vi "PH_gentec_Powermeter.Action open connection.vi"(0 "VI in":refnum<vi>, 5 "error in (no error)":errorcluster) -> (14 "VI out":refnum<vi>, 19 "error out":errorcluster)   [LabVIEW 2014, in "PH_gentec_Powermeter.lvlib"]
uses:
  PH_gentec_Powermeter.lvlib
  PH_Powermeter_BaseClass/PH_Powermeter_BaseClass.State.ctl
  PH_Powermeter_BaseClass/PH_Powermeter_BaseClass.lvlib
  non_GPL/instr.lib/gentec-SOLO-PE/gentec-SOLO-PE - Driver.lvlib
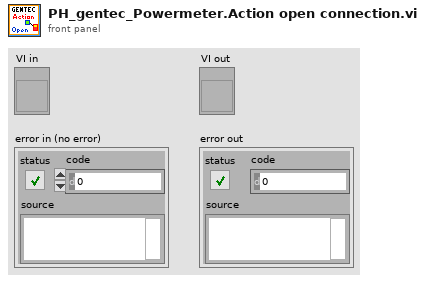
[diagram p1: front panel]
types:
  T1 = typedef "PH_Powermeter_BaseClass.lvlib/PH_Powermeter_BaseClass.State.ctl" = enum32{"off", "operating", "opened", "checked", "connected", "Sets to change", "running"}
  T2 = typedef "PH_Powermeter_BaseClass.lvlib/PH_Powermeter_BaseClass.i attribute.ctl" = cluster{"GUI References":T3, "Connection":T4, "Head Attributes":T5, "VISA resource":refnum<visa-resource-name>, "Energy":T6, "Service ID Energy":i32, "Wanted Settings":T7, "Current Settings":T7}
  T3 = typedef "PH_Powermeter_BaseClass.lvlib/PH_Powermeter_BaseClass.GUI Refs.ctl" = cluster{"Head Attributes":refnum<vi>, "Energy":refnum<vi>, "Connection":refnum<vi>, "VISA Resource":refnum<vi>, "Energy evolution":refnum<vi>, "Scaling Factor":refnum<vi>, "Range":refnum<vi>, "Wavelength":refnum<vi>, "Trigger Level":refnum<vi>, "Wanted Settings":refnum<vi>, "Current Settings":refnum<vi>}
  T4 = typedef "PH_Powermeter_BaseClass.lvlib/PH_Powermeter_BaseClass.Connection.ctl" = cluster{"failed checks":i8, "Timeout":bool, "Data read":string, "Failure":bool, "Error":bool, "State":T1}
  T5 = typedef "PH_Powermeter_BaseClass.lvlib/PH_Powermeter_BaseClass.Head Attributes.ctl" = cluster{"Instrument Type":string, "Head Version":string, "Head Name":string, "Serial Number":string, "Firmware":string, "Sensor Type":string, "MinimumRange":u32, "Maximum Range":u32, "Min Wavelength":i32, "Max Wavelength":i32}
  T6 = typedef "PH_Powermeter_BaseClass.lvlib/PH_Powermeter_BaseClass.Energy.ctl" = cluster{"current Value":dbl, "unscaled":dbl, "Scaling Factor":dbl}
  T7 = typedef "PH_Powermeter_BaseClass.lvlib/PH_gentec_BaseClass.Head Settings.ctl" = cluster{"Trigger Level":dbl, "Wavelength":u32, "Range":u32}
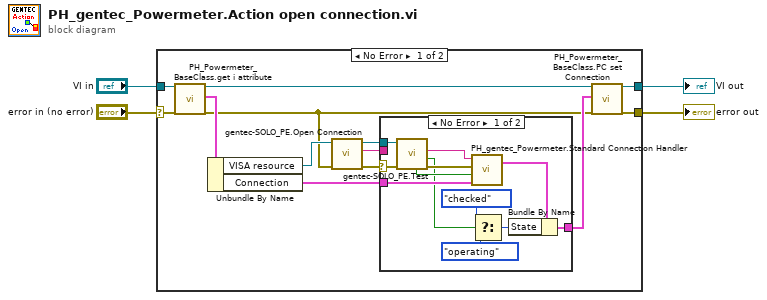
[diagram p0: block diagram]
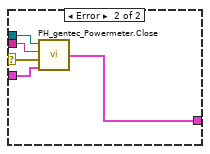
[diagram p2: hidden frame]
diagram:
  n1 = case shown="No Error" "error in (no error)" {
    selector: "error in (no error)" -> [w5 w35]
    tunnel: [w17 w35] -> w4
    tunnel: [w16 w36] -> w3
    tunnel: "VI in" -> [w11 w36]
    frame No Error {
      n2 = call "PH_Powermeter_BaseClass.get i attribute.vi"("i ref in"=w11, "error in (no error)"=w5) -> ("i ref out"=w9:refnum<vi>, "i attribute"=w12:T2, "error out"=w10:errorcluster)  [unwired: 15 in]
      n3 = Unbundle By Name(w12) -> ("VISA resource"=w15:refnum<visa-resource-name>, "Connection"=w14:T4)
      n4 = call "gentec-SOLO_PE.Open Connection.vi"("error in"=w10, "VISA resource name in"=w15) -> ("error out"=w6:errorcluster, "Error"=w8:string, "VISA resource name out"=w7:refnum<visa-resource-name>)  [unwired: 3 in]
      n5 = case shown="No Error" w6 {
        selector: w6 -> [w28 w33]
        tunnel: w7 -> [w29 w34]
        tunnel: w8 -> [_ w32]
        tunnel: w14 -> [w22 w31]
        tunnel: [w23 w30] -> w13
        frame No Error {
          n6 = call "gentec-SOLO_PE.Test.vi"("error in (no error)"=w28, "VISA Refnum in"=w29) -> ("error out"=w25:errorcluster, "Acknoledged?"=w21:bool, "Error"=w27:string, "Timeout"=w26:bool)  [unwired: 5 in, 1 out]
          n7 = call "PH_gentec_Powermeter.Standard Connection Handler.vi"("Connection in"=w22, "Timeout"=w26, "Device Error"=w25, "Error"=w27) -> ("Connection out"=w24:T4)  [unwired: 1 out]
          n8 = Select(t=PH_Powermeter_BaseClass.State."checked" ("State"), s=w21, f=PH_Powermeter_BaseClass.State."operating" ("State")) -> (s? t:f=w20:T1)
          n9 = Bundle By Name(cluster=w24, "State"=w20) -> (w23:T4)
        }
        frame Error {
          n10 = call "PH_gentec_Powermeter.Close.vi"("Connection in"=w31, "Device Error in"=w33, "Error Message"=w32, "VISA Refnum in"=w34) -> ("Connection out"=w30:T4)
        }
      }
      n11 = call "PH_Powermeter_BaseClass.PC set Connection.vi"("VI in"=w9, "Connection"=w13, "error in (no error)"=w10) -> ("VI out"=w16:refnum<vi>, "error out"=w17:errorcluster)  [unwired: 15 in]
    }
    frame Error {
    }
  }
  "error out" <- w4
  "VI out" <- w3
